vi "AP Main.vi"() -> ()   [LabVIEW 2012]
uses:
  <userlib>/H_Utilities/myDAQ_State.ctl
  Controls/Sheet Colors.ctl
  Controls/Quiz Question.ctl
  Controls/Quiz Solution.ctl
  Spreadsheet/Controls/Spreadsheet Commands.ctl
  Controls/Quiz Mode.ctl
  <vilib>/Utility/sysdir.llb/System Directory Type.ctl
  <vilib>/Platform/browser.llb/Open URL in Default Browser (string).vi
  <userlib>/H_Utilities/myDAQmx/myDAQmx Create Channel/Create myDAQ AI.vi
  <userlib>/H_Utilities/myDAQmx/myDAQmx Create Channel/Create myDAQ DO.vi
  <userlib>/H_Utilities/myDAQmx/myDAQmx Read/myDAQmx Read Analog Value.vi
  <userlib>/H_Utilities/myDAQmx/myDAQmx Read/myDAQmx Read Analog Waveforms.vi
  <userlib>/H_Utilities/myDAQmx/myDAQmxWrite/myDAQmx Write Digital - 1 Chan.vi
panel:
  in  "Quiz Atempts":i32=2
  out "Quiz Questions":i32
  in  "Sheet Colors":T1={"Header Color"=16758784, "Header Font Color"=0, "Font Color"=0, "Clear Color"=16777225, "Alt Clear Color"=15000804}
  in  "AG Page Buttons":enum32{"Page 1", "Page 2", "Page 3", "Page 4"}(radio)
  in  "Exit":bool
  in  "LabVIEW":bool
  in  "Report Issue":bool
  out "Error Out":errorcluster
  out "Event Loop":i32
  out "DAQ Loop":i32
  out "Active State":T2
  in  "AG Pages":enum32{"Page 1", "Page 2", "Page 3", "Page 4"}(tab)
  in  "Explore":bool
  out "Connected":bool
  in  "AG Tab Buttons":enum32{"Tab1", "Tab2", "Tab3"}(radio)
  in  "AG Tabs":enum32{"Tab 1", "Tab 2", "Tab 3"}(tab)
  in  "Configure":bool
  out "Value":dbl(slide) scale=-10.0..10.0
  in  "Measure":bool
  out "Analog Input 0":dbl(knob) scale=-10.0..10.0 scale format="%#.3g"
  in  "DO":bool
  out "Waveform Chart":waveform(dbl)(graph)
  in  "Log to Table":bool
  in  "Event Name":string="Event 1"
  out "Elapsed Time":dbl format="%.2gs"
  in  "Spreadsheet":i32[](listbox)
  in  "Copy":bool
  in  "Clear Sheet":bool
  in  "Save as .csv":bool
  in  "Next Question":bool
  in  "Previous Question":bool
  in  "Grade":bool
  out "Grade String":string
  in  "Problem3":T3={"ProblemNum"=0, "Problem Type"={"Text"="", "Image"=bytes[0], "Text&Image"={"Text (&Image)"="", "Image (&text)"=bytes[0]}}, "Solution Type"={"Numeric"=0.0, "Text"="", "Multi"={"A"=TRUE, "B"=FALSE, "C"=FALSE, "D"=FALSE, "E"=FALSE}, "Radio"=enum."A", "True/False"=enum."True", "Short Answer"=""}, "Answer Color"=0}
  in  "Problem2":T3={"ProblemNum"=0, "Problem Type"={"Text"="", "Image"=bytes[0], "Text&Image"={"Text (&Image)"="", "Image (&text)"=bytes[0]}}, "Solution Type"={"Numeric"=0.0, "Text"="", "Multi"={"A"=TRUE, "B"=FALSE, "C"=FALSE, "D"=FALSE, "E"=FALSE}, "Radio"=enum."A", "True/False"=enum."True", "Short Answer"=""}, "Answer Color"=0}
  in  "Problem1":T3={"ProblemNum"=0, "Problem Type"={"Text"="", "Image"=bytes[0], "Text&Image"={"Text (&Image)"="", "Image (&text)"=bytes[0]}}, "Solution Type"={"Numeric"=0.0, "Text"="", "Multi"={"A"=TRUE, "B"=FALSE, "C"=FALSE, "D"=FALSE, "E"=FALSE}, "Radio"=enum."A", "True/False"=enum."True", "Short Answer"=""}, "Answer Color"=0}
  in  "Problem0":T3={"ProblemNum"=0, "Problem Type"={"Text"="", "Image"=bytes[0], "Text&Image"={"Text (&Image)"="", "Image (&text)"=bytes[0]}}, "Solution Type"={"Numeric"=0.0, "Text"="", "Multi"={"A"=TRUE, "B"=FALSE, "C"=FALSE, "D"=FALSE, "E"=FALSE}, "Radio"=enum."A", "True/False"=enum."True", "Short Answer"=""}, "Answer Color"=0}
  in  "Quiz Scrollbar":i32(c297)
  # "Lab Title"
  # "#update\nIf you change this remeber to set as default"
  # "Getting Started Instructions"
  # "1. Connect myDAQ to this computer.\n\n2. Connect the circuit as shown here."
  # "1. Calibrate your device"
  # "1. Read Signal"
  # "Spreadsheet Title"
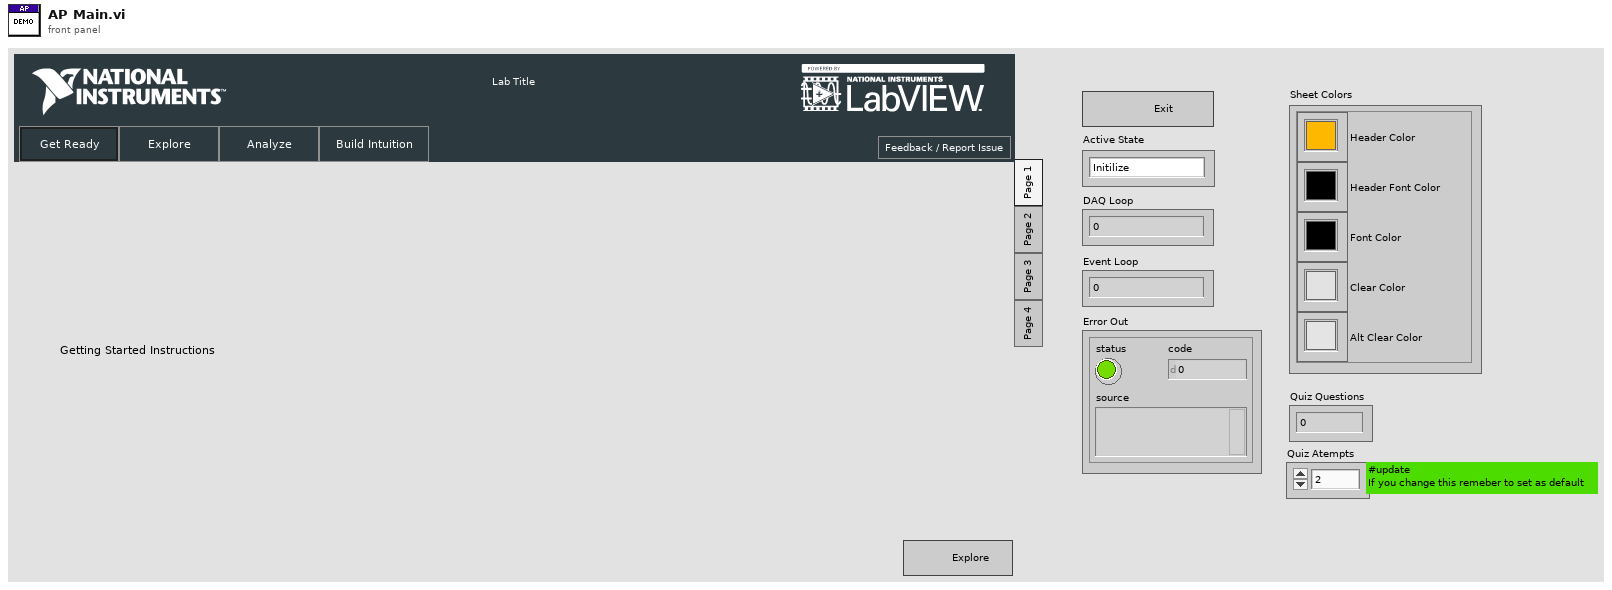
[diagram p1: front panel]
types:
  T1 = typedef "Sheet Colors.ctl" = cluster{"Header Color":u32, "Header Font Color":u32, "Font Color":u32, "Clear Color":u32, "Alt Clear Color":u32}
  T2 = typedef "myDAQ_State.ctl" = enum16{"Initilize", "Connect", "Calibrate", "Communicate", "Wait", "Disconnect", "Error", "Close"}
  T3 = typedef "Quiz Question.ctl" = cluster{"ProblemNum":i32, "Problem Type":cluster{"Text":string, "Image":picture, "Text&Image":cluster{"Text (&Image)":string, "Image (&text)":picture}}, "Solution Type":T4, "Answer Color":u32}
  T4 = typedef "Quiz Solution.ctl" = cluster{"Numeric":dbl, "Text":string, "Multi":cluster{"A":bool, "B":bool, "C":bool, "D":bool, "E":bool}, "Radio":enum32{"No Selection", "A", "B", "C", "D", "E"}, "True/False":enum32{"No Selection", "True", "False"}, "Short Answer":string}
  T5 = enum8{"Enabled", "Disabled", "Disabled and Grayed Out"}
  T6 = typedef "Spreadsheet Commands.ctl" = enum16{"Init", "Clear", "Add", "Mass Add", "Delete Row", "Format Colors"}
  T7 = typedef "Quiz Info.ctl" = cluster{"Question Type":enum16{"Text", "Image", "Text&Image"}, "Solution Type":enum16{"Number", "Text", "MultiChoice", "Radio", "T/F", "Paragraph"}, "Question":cluster{"Text":string, "Image":picture}, "Solution":cluster{"Numeric":cluster{"Min":dbl, "Max":dbl, "Sig Figs":i32, "Sig Figs?":bool}, "Text":string, "True/False":bool, "MultiSelect":cluster{"A":bool, "B":bool, "C":bool, "D":bool, "E":bool}, "MultiText":string[], "Text Case Match":bool}, "Stored Solution":T4, "Button Color":u32}
  T8 = enum32{"invalid app kind", "Development System", "Run Time System", "Student Edition", "Embedded LabVIEW", "Evaluation", "Custom"}
  T9 = typedef "Quiz Mode.ctl" = enum16{"Update", "Store Solution", "Grade"}
  T10 = typedef "System Directory Type.ctl" = i32
  T11 = typedef "LVPoint32TypeDef.ctl" = cluster{"Horizontal":i32, "Vertical":i32}
  T12 = typedef "LVRowAndColumnTypeDef.ctl" = cluster{"Row":i32, "Column":i32}
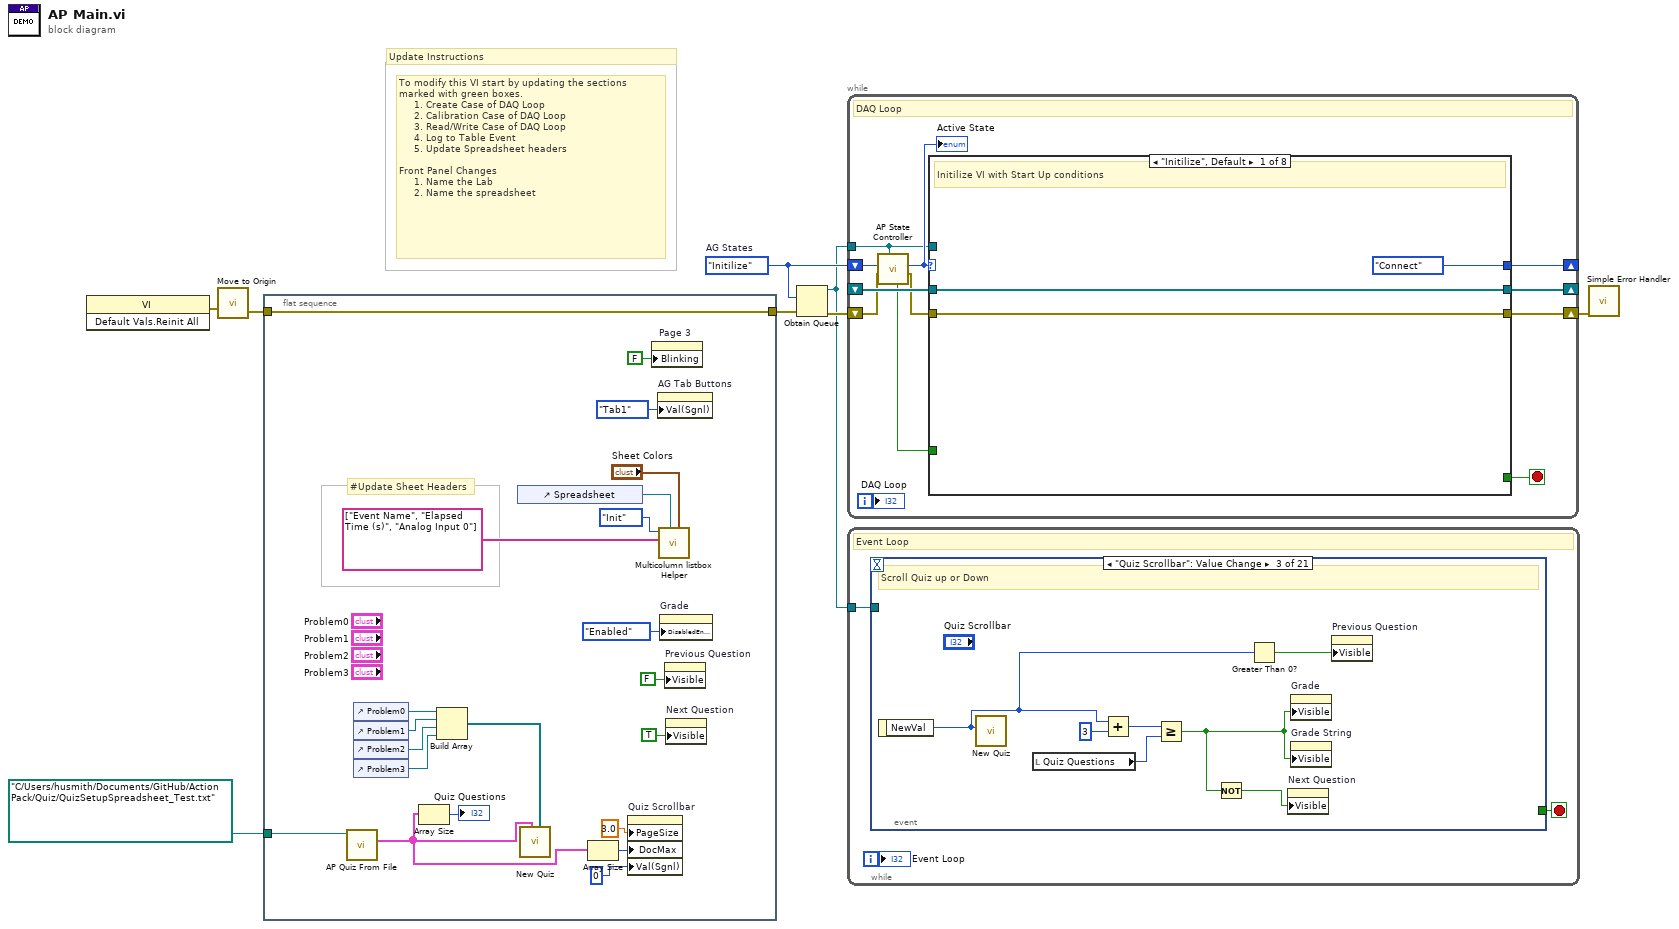
[diagram p0: block diagram]
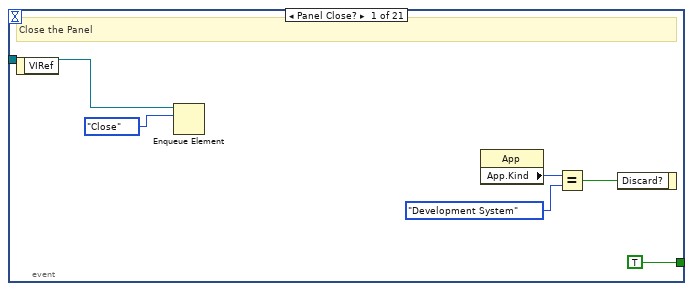
[diagram p2: hidden frame]
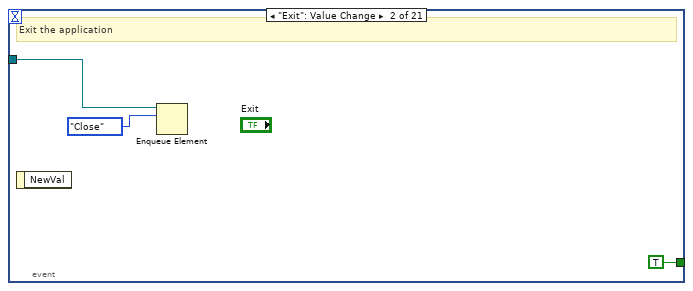
[diagram p3: hidden frame]
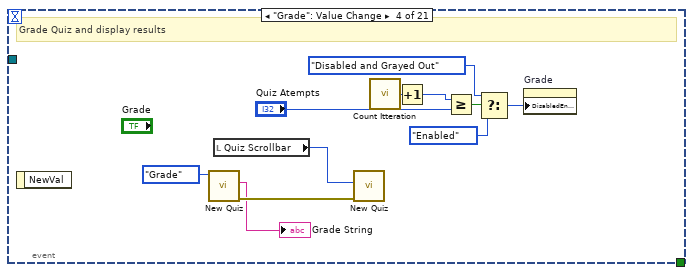
[diagram p4: hidden frame]
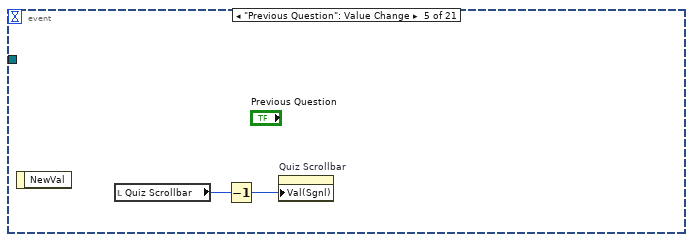
[diagram p5: hidden frame]
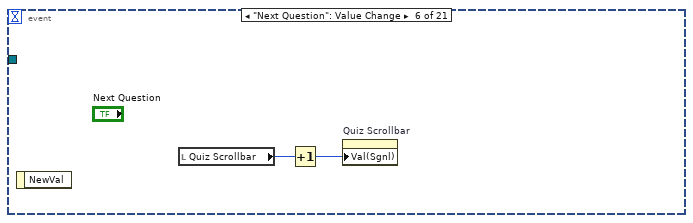
[diagram p6: hidden frame]
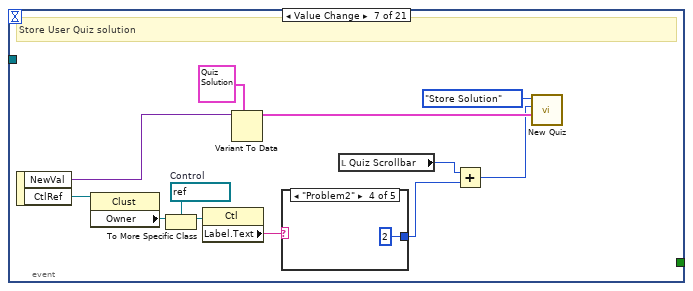
[diagram p7: hidden frame]
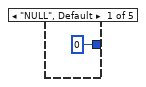
[diagram p8: hidden frame]
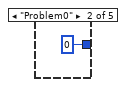
[diagram p9: hidden frame]
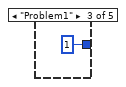
[diagram p10: hidden frame]
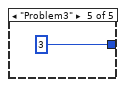
[diagram p11: hidden frame]
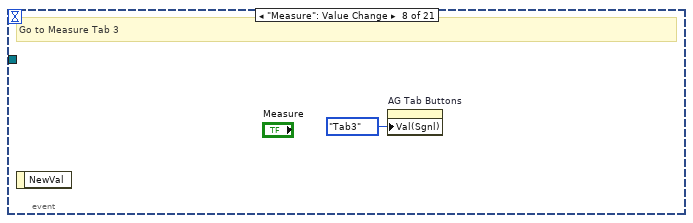
[diagram p12: hidden frame]
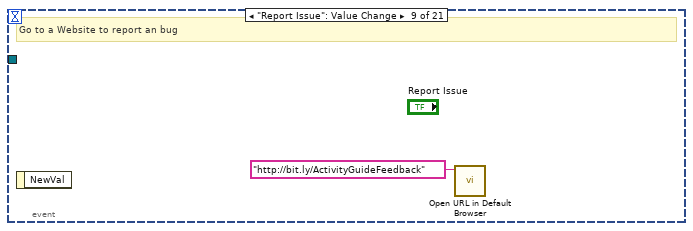
[diagram p13: hidden frame]
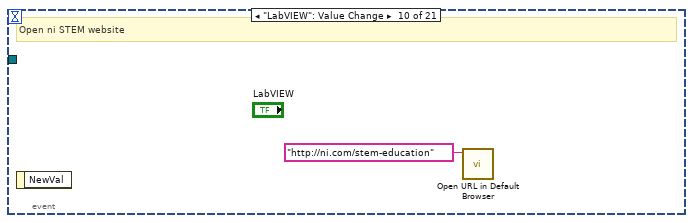
[diagram p14: hidden frame]
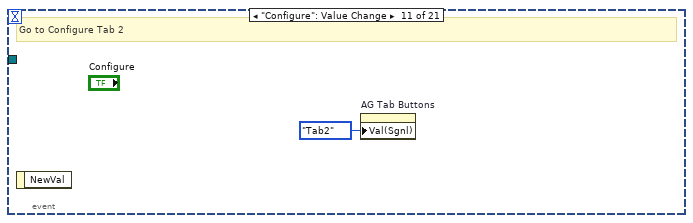
[diagram p15: hidden frame]
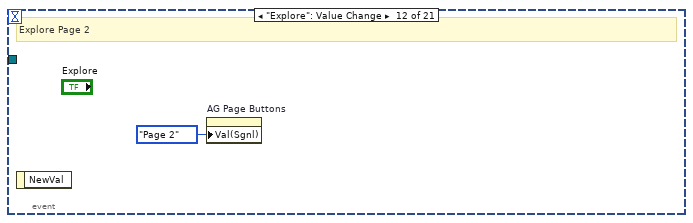
[diagram p16: hidden frame]
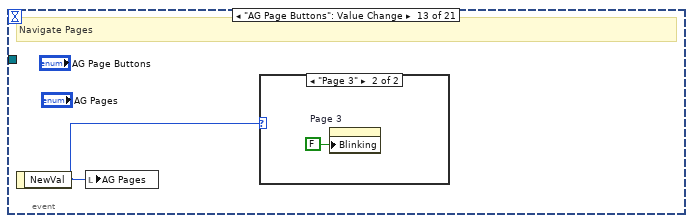
[diagram p17: hidden frame]
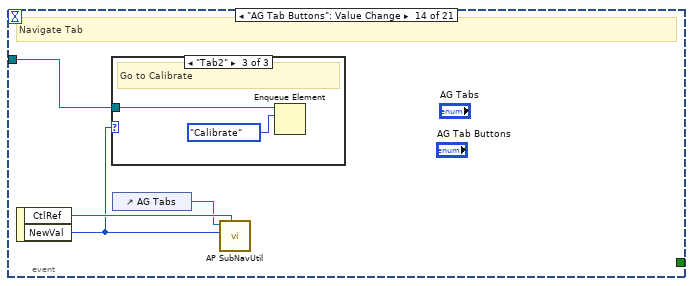
[diagram p19: hidden frame]
diagram:
  w8 = myDAQ_State."Initilize"  # AG States
  # "To modify this VI start by updating the sections marked with green boxes.\n     1. Create Case of DAQ Loop\n     2. Calibration Case of DAQ Loop\n     3. Read/Write Case of DAQ Loop\n     4. Log to Table Event\n     5. Update Spreadsheet headers\n\nFront Panel Changes\n     1. Name the Lab\n     2. Name the spreadsheet"
  # "Update Instructions"
  n1 = invoke class="VI" method="Default Vals.Reinit All"() -> (error out=w2:errorcluster)  [unwired: 3 in, 2 out]
  n2 = call "Move to Origin.vi"("Error In"=w2) -> ("Error Out"=w4:errorcluster)  [unwired: 2 in]
  n3 = flat-sequence {
    tunnel: w4 -> [w29]
    tunnel: [w29] -> w3
    tunnel: path "C:/Users/husmith/Documents/GitHub/Action Pack/Quiz/QuizSetupSpreadsheet_Test.txt" ("file path (dialog if empty)") -> [w14]
    frame #0 {
      # "#Update Sheet Headers"
      n4 = call "AP Quiz From File.vi"("file path (dialog if empty)"=w14) -> ("Question Array Out"=w11:T7[])  [unwired: 8 in, 2 out]
      n5 = control-ref of="Problem0"() -> (w22:refnum<vi>)
      n6 = control-ref of="Problem1"() -> (w21:refnum<vi>)
      n7 = control-ref of="Problem2"() -> (w20:refnum<vi>)
      n8 = control-ref of="Problem3"() -> (w19:refnum<vi>)
      n9 = Array Size(array=w11) -> (size(s)=→"Quiz Questions":i32)
      n10 = Build Array(w22, w21, w20, w19) -> (w18:refnum<vi>[])
      n11 = control-ref of="Spreadsheet"() -> (w24:refnum<vi>)
      n12 = call "New Quiz.vi"("Prob Ref"=w18, "Quiz Data"=w11) -> ()  [unwired: 8 in, 2 out]
      n13 = Array Size(array=w11) -> (size(s)=w17:i32)
      n14 = property on="Quiz Scrollbar" class="Scroll (strict)"("PageSize"=3.0 ("Page Size"), "DocMax"=w17, "Val(Sgnl)"=0 ("Value (Signaling)")) -> ()  [unwired: 2 in, 2 out]
      n15 = property on="Page 3" class="Bool (strict)"("Blinking"=FALSE) -> ()  [unwired: 2 in, 2 out]
      n16 = property on="AG Tab Buttons" class="RadioBtnsControl (strict)"("Val(Sgnl)"=enum32{"Tab1", "Tab2", "Tab3"}."Tab1" ("Value (Signaling)")) -> ()  [unwired: 2 in, 2 out]
      n17 = call "Multicolumn listbox Helper.vi"("Sheet Colors"="Sheet Colors", "Multicolumn Ref"=w24, "Data"=string[] ["Event Name", "Elapsed Time (s)", "Analog Input 0"], "Action (add default)"=Spreadsheet_Commands."Init") -> ()  [unwired: 7 in, 1 out]
      n18 = property on="Grade" class="Bool"("DisabledEnum"=T5."Enabled" ("Disabled")) -> ()  [unwired: 2 in, 2 out]
      n19 = property on="Previous Question" class="Bool"("Visible"=FALSE) -> ()  [unwired: 2 in, 2 out]
      n20 = property on="Next Question" class="Bool"("Visible"=TRUE) -> ()  [unwired: 2 in, 2 out]
    }
  }
  n21 = Obtain Queue(element data type=w8, error in (no error)=w3) -> (queue out=w6:refnum<queue>, error out=w7:errorcluster)  [unwired: 3 in, 1 out]
  n22 = while {
    shift-right: [w41] -> _
    shift-left: _ -> [w39]
    shift-right: [w34] -> _
    shift-left: w8 -> [w38]
    tunnel: w6 -> [w31]
    shift-right: [w40] -> w5
    shift-left: w7 -> [w37]
    i -> [w30]
    stop <- w32 stop-if-true
    # "DAQ Loop"
    n23 = call "AP State Controller.vi"("queue Ref"=w31, "Error In"=w37, "Default State"=w38) -> ("Error Out"=w36:errorcluster, "State Out"=w33:T2, "New State"=w35:bool)  [unwired: 6 in]
    "Active State" <- w33
    n24 = case shown="\"Initilize\", Default" w33 {
      tunnel: [w44 w46 w66 w75 w83 w95 w102 w111] -> w41
      tunnel: [w42 w47 w67 w76 w90 w94 w101 w110] -> w40
      tunnel: w39 -> [w44 w62 w69 w82 w87 w97 w104 w109]
      tunnel: w36 -> [w42 w61 w68 w81 w86 w96 w103 w108]
      tunnel: w35 -> [_ w58 _ _ _ _ _ _]
      tunnel: [myDAQ_State."Connect" ("AG States") w52 myDAQ_State."Calibrate" ("AG States") myDAQ_State."Communicate" ("AG States") w84 myDAQ_State."Wait" ("AG States") w98 myDAQ_State."Close" ("AG States")] -> w34
      tunnel: [_ _ _ _ _ _ _ TRUE] -> w32
      tunnel: w31 -> [_ _ _ _ w91 _ _ _]
      frame "Initilize", Default {
        # "Initilize VI with Start Up conditions"
      }
      frame "Connect" {
        # "#Update Create DAQ Tasks"
        # "Connect to myDAQmx Tasks"
        n25 = call <userlib>:"myDAQmx Safe Clear.vi"("error in (no error)"=w61, "task array in"=w62) -> ("error out"=w60:errorcluster, "task array out"=w63:refnum<k21>[])  [unwired: 8 in]
        n26 = Select(t=u32 0 ("milliseconds to wait"), s=w58, f=u32 250 ("milliseconds to wait")) -> (s? t:f=w55:u32)
        n27 = Wait (ms)(milliseconds to wait=w55) -> ()  [unwired: 1 out]
        n28 = call-poly <userlib>:"myDAQmx Create Channel.vi"("samples per channel(100)"=1, "error in (no error)"=w60, "physical channels (ai0:1)"=tag "myDAQ1/ai0:1", "task array in (none)"=w63) -> ("error out"=w49:errorcluster, "task array out"=w48:refnum<k21>[])  [unwired: 6 in]
        n29 = call-poly <userlib>:"myDAQmx Create Channel.vi"("error in (no error)"=w49, "task array in (none)"=w48) -> ("error out"=w47:errorcluster, "task array out"=w46:refnum<k21>[])  [unwired: 8 in]
        n30 = Unbundle By Name(w47) -> ("status"=w51:bool)
        n31 = Select(t=myDAQ_State."Connect" ("AG States"), s=w47, f=myDAQ_State."Wait" ("AG States")) -> (s? t:f=w52:T2)
        n32 = Not(x=w51) -> (.not. x?=→"Connected":bool)
      }
      frame "Calibrate" {
        # "#Update Calibrate"
        # "Calibrate DAQ Tasks"
        n33 = call-poly <userlib>:"myDAQmx Read.vi"("error in (no error)"=w68, "task array in"=w69) -> ("error out"=w67:errorcluster, "value 0"=→"Value":dbl, "task array out"=w66:refnum<k21>[])  [unwired: 6 in, 1 out]
        n34 = Wait Until Next ms Multiple(millisecond multiple=u32 20) -> ()  [unwired: 1 out]
      }
      frame "Communicate" {
        # "#Update Read /Write DAQ & Analyze"
        # "Read / Write myDAQmx Tasks Here & perform analysis"
        n35 = call-poly <userlib>:"myDAQmx Read.vi"("error in (no error)"=w81, "# of samples per channel (-1)"=1, "task array in"=w82) -> ("error out"=w77:errorcluster, "waveform 1"=w72:waveform(dbl), "task array out"=w78:refnum<k21>[])  [unwired: 2 in, 4 out]
        "Waveform Chart" <- w72
        "Analog Input 0" <- w72
        n36 = call "Extract M-S from Timestamp.vi"("Waveform"=w72) -> ("Elapsed Time (s)"=→"Elapsed Time":dbl)  [unwired: 9 in, 1 out]
        n37 = call-poly <userlib>:"myDAQmx Write.vi"("error in (no error)"=w77, "value (F)"="DO", "task array in"=w78) -> ("error out"=w76:errorcluster, "task array out"=w75:refnum<k21>[])  [unwired: 7 in]
        n38 = Wait Until Next ms Multiple(millisecond multiple=u32 20) -> ()  [unwired: 1 out]
      }
      frame "Wait" {
        # "Wait for New Command in State Queue"
        n39 = call <userlib>:"myDAQmx Stop Task.vi"("error In"=w86, "task array in"=w87) -> ("Error Out"=w88:errorcluster, "task array out"=w89:refnum<k21>[])  [unwired: 8 in]
        n40 = call <userlib>:"myDAQmx Handle Errors.vi"("Error In"=w88, "Task Array In"=w89) -> ("Error Out"=w85:errorcluster, "Task Array Out"=w83:refnum<k21>[])  [unwired: 6 in, 2 out]
        n41 = Preview Queue Element(queue=w91, error in (no error)=w85) -> (element=w84:T2, error out=w90:errorcluster)  [unwired: 1 in, 2 out]
      }
      frame "Disconnect" {
        # "Disconnect from DAQ device"
        n42 = call <userlib>:"myDAQmx Safe Clear.vi"("error in (no error)"=w96, "task array in"=w97) -> ("error out"=w94:errorcluster, "task array out"=w95:refnum<k21>[])  [unwired: 8 in]
        n43 = local write "Connected"(FALSE ("Connected")) -> ()
      }
      frame "Error" {
        # "Error Found, Handle and Continue"
        n44 = call <userlib>:"myDAQmx Handle Errors.vi"("Error In"=w103, "Task Array In"=w104) -> ("Error Out"=w101:errorcluster, "Task Array Out"=w102:refnum<k21>[])  [unwired: 6 in, 2 out]
        n45 = Select(t=myDAQ_State."Close" ("AG States"), s=w101, f=myDAQ_State."Connect" ("AG States")) -> (s? t:f=w98:T2)
        "Error Out" <- w103
      }
      frame "Close" {
        n46 = local write "Connected"(FALSE ("Connected")) -> ()
        n47 = property on="Exit" class="Bool (strict)"("Val(Sgnl)"=TRUE ("Connected")) -> ()  [unwired: 2 in, 2 out]
        n48 = call <userlib>:"myDAQmx Safe Clear.vi"("error in (no error)"=w108, "task array in"=w109) -> ("error out"=w110:errorcluster, "task array out"=w111:refnum<k21>[])  [unwired: 8 in]
      }
    }
    "DAQ Loop" <- w30
  }
  n49 = while {
    tunnel: w6 -> [w115]
    i -> [w113]
    stop <- w114 stop-if-true
    # "Event Loop"
    n50 = event shown="[2] \"Quiz Scrollbar\": Value Change" {
      selector: _ -> [_ _ _ _ _ _ _ _ _ _ _ _ _ _ _ _ _ _ _ _ _]
      dyn-events: _ -> [_ _ _ _ _ _ _ _ _ _ _ _ _ _ _ _ _ _ _ _ _]
      timeout: _ -> [_ _ _ _ _ _ _ _ _ _ _ _ _ _ _ _ _ _ _ _ _]
      tunnel: w115 -> [w121 w124 _ _ _ _ _ _ _ _ _ _ _ w171 _ _ _ _ _ _ _]
      tunnel: [TRUE TRUE _ _ _ _ _ _ _ _ _ _ _ _ _ _ _ _ _ _ _] -> w114
      event Panel Close? {
        # "Close the Panel"
        n51 = event-data() -> ()  [unwired: 1 in, 1 out]
        n52 = Enqueue Element(queue=w121, element=myDAQ_State."Close") -> ()  [unwired: 2 in, 3 out]
        n53 = property class="App"() -> ("App.Kind"=w118:T8)  [unwired: 2 in, 2 out]
        n54 = Equal?(x=w118, y=T8."Development System" ("Application:Kind")) -> (x = y?=w116:bool)
        n55 = event-data("Discard?"=w116) -> ()  [unwired: 1 in, 1 out]
      }
      event "Exit": Value Change {
        # "Exit the application"
        n56 = event-data() -> ()  [unwired: 1 in, 1 out]
        n57 = Enqueue Element(queue=w124, element=myDAQ_State."Close") -> ()  [unwired: 2 in, 3 out]
      }
      event "Quiz Scrollbar": Value Change {
        # "Scroll Quiz up or Down"
        n58 = event-data() -> ("NewVal"=w128:i32)  [unwired: 1 in]
        n59 = call "New Quiz.vi"("Index"=w128) -> ()  [unwired: 9 in, 2 out]
        n60 = local read "Quiz Questions"() -> (w129:i32)
        n61 = Add(x=w128, y=3) -> (x+y=w130:i32)
        n62 = Greater Or Equal?(x=w130, y=w129) -> (x >= y?=w126:bool)
        n63 = Not(x=w126) -> (.not. x?=w125:bool)
        n64 = Greater Than 0?(x=w128) -> (x > 0?=w127:bool)
        n65 = property on="Next Question" class="Bool"("Visible"=w125) -> ()  [unwired: 2 in, 2 out]
        n66 = property on="Grade" class="Bool"("Visible"=w126) -> ()  [unwired: 2 in, 2 out]
        n67 = property on="Grade String" class="Str"("Visible"=w126) -> ()  [unwired: 2 in, 2 out]
        n68 = property on="Previous Question" class="Bool"("Visible"=w127) -> ()  [unwired: 2 in, 2 out]
      }
      event "Grade": Value Change {
        # "Grade Quiz and display results"
        n69 = event-data() -> ()  [unwired: 1 in, 1 out]
        n70 = call "New Quiz.vi"("Mode"=Quiz_Mode."Grade") -> ("Error Out"=w141:errorcluster, "Grade String"=→"Grade String":string)  [unwired: 9 in]
        n71 = local read "Quiz Scrollbar"() -> (w140:i32)
        n72 = call "New Quiz.vi"("Error In"=w141, "Index"=w140) -> ()  [unwired: 8 in, 2 out]
        n73 = call "Count Itteration.vi"() -> ("Itteration"=w138:i32)  [unwired: 7 in, 1 out]
        n74 = Increment(x=w138) -> (x+1=w132:i32)
        n75 = Greater Or Equal?(x=w132, y="Quiz Atempts") -> (x >= y?=w136:bool)
        n76 = Select(t=T5."Disabled and Grayed Out" ("Disabled"), s=w136, f=T5."Enabled" ("Disabled")) -> (s? t:f=w133:T5)
        n77 = property on="Grade" class="Bool"("DisabledEnum"=w133) -> ()  [unwired: 2 in, 2 out]
      }
      event "Previous Question": Value Change {
        n78 = event-data() -> ()  [unwired: 1 in, 1 out]
        n79 = local read "Quiz Scrollbar"() -> (w144:i32)
        n80 = Decrement(x=w144) -> (x-1=w143:i32)
        n81 = property on="Quiz Scrollbar" class="Scroll (strict)"("Val(Sgnl)"=w143) -> ()  [unwired: 2 in, 2 out]
      }
      event "Next Question": Value Change {
        n82 = event-data() -> ()  [unwired: 1 in, 1 out]
        n83 = local read "Quiz Scrollbar"() -> (w146:i32)
        n84 = Increment(x=w146) -> (x+1=w145:i32)
        n85 = property on="Quiz Scrollbar" class="Scroll (strict)"("Val(Sgnl)"=w145) -> ()  [unwired: 2 in, 2 out]
      }
      event Value Change {
        w152 = refnum<vi> refnum  # Control
        # "Store User Quiz solution"
        n86 = event-data() -> ("NewVal"=w158:variant, "CtlRef"=w155:refnum<vi>)  [unwired: 1 in]
        n87 = property class="Clust"(reference=w155) -> ("Owner"=w154:refnum<vi>)  [unwired: 1 in, 2 out]
        n88 = To More Specific Class(target class=w152, reference=w154) -> (specific class reference=w153:refnum<vi>)  [unwired: 1 in, 1 out]
        n89 = property class="Ctl"(reference=w153) -> ("Label.Text"=w151:string)  [unwired: 1 in, 2 out]
        n90 = Variant To Data(type=T4 {"Numeric"=0.0, "Text"="", "Multi"={"A"=FALSE, "B"=FALSE, "C"=FALSE, "D"=FALSE, "E"=FALSE}, "Radio"=enum."No Selection", "True/False"=enum."No Selection", "Short Answer"=""} ("Quiz Solution"), Variant=w158) -> (data=w156:T4)  [unwired: 1 in, 1 out]
        n91 = case shown="\"Problem2\"" w151 {
          tunnel: [0 0 1 2 3] -> w149
          frame "NULL", Default {
          }
          frame "Problem0" {
          }
          frame "Problem1" {
          }
          frame "Problem2" {
          }
          frame "Problem3" {
          }
        }
        n92 = local read "Quiz Scrollbar"() -> (w150:i32)
        n93 = Add(x=w150, y=w149) -> (x+y=w148:i32)
        n94 = call "New Quiz.vi"("Quiz Solution"=w156, "Index"=w148, "Mode"=Quiz_Mode."Store Solution") -> ()  [unwired: 7 in, 2 out]
      }
      event "Measure": Value Change {
        # "Go to Measure Tab 3"
        n95 = event-data() -> ()  [unwired: 1 in, 1 out]
        n96 = property on="AG Tab Buttons" class="RadioBtnsControl (strict)"("Val(Sgnl)"=enum32{"Tab1", "Tab2", "Tab3"}."Tab3" ("Value (Signaling)")) -> ()  [unwired: 2 in, 2 out]
      }
      event "Report Issue": Value Change {
        # "Go to a Website to report an bug"
        n97 = event-data() -> ()  [unwired: 1 in, 1 out]
        n98 = call-poly <vilib>:"Open URL in Default Browser.vi"("URL"="http://bit.ly/ActivityGuideFeedback") -> ()  [unwired: 5 in, 2 out]
      }
      event "LabVIEW": Value Change {
        # "Open ni STEM website"
        n99 = event-data() -> ()  [unwired: 1 in, 1 out]
        n100 = call-poly <vilib>:"Open URL in Default Browser.vi"("URL"="http://ni.com/stem-education") -> ()  [unwired: 5 in, 2 out]
      }
      event "Configure": Value Change {
        # "Go to Configure Tab 2"
        n101 = event-data() -> ()  [unwired: 1 in, 1 out]
        n102 = property on="AG Tab Buttons" class="RadioBtnsControl (strict)"("Val(Sgnl)"=enum32{"Tab1", "Tab2", "Tab3"}."Tab2" ("Value (Signaling)")) -> ()  [unwired: 2 in, 2 out]
      }
      event "Explore": Value Change {
        # "Explore Page 2"
        n103 = event-data() -> ()  [unwired: 1 in, 1 out]
        n104 = property on="AG Page Buttons" class="RadioBtnsControl (strict)"("Val(Sgnl)"=enum32{"Page 1", "Page 2", "Page 3", "Page 4"}."Page 2" ("Value (Signaling)")) -> ()  [unwired: 2 in, 2 out]
      }
      event "AG Page Buttons": Value Change {
        # "Navigate Pages"
        n105 = event-data() -> ("NewVal"=w169:enum32{"Page 1", "Page 2", "Page 3", "Page 4"})  [unwired: 1 in]
        n106 = local write "AG Pages"(w169) -> ()
        n107 = case shown="\"Page 3\"" w169 {
          frame "Page 1", Default {
          }
          frame "Page 3" {
            n108 = property on="Page 3" class="Bool (strict)"("Blinking"=FALSE) -> ()  [unwired: 2 in, 2 out]
          }
        }
      }
      event "AG Tab Buttons": Value Change {
        # "Navigate Tab"
        n109 = event-data() -> ("CtlRef"=w174:refnum<vi>, "NewVal"=w172:enum32{"Tab1", "Tab2", "Tab3"})  [unwired: 1 in]
        n110 = case shown="\"Tab2\"" w172 {
          tunnel: w171 -> [_ w175 w177]
          frame "Tab1", Default {
          }
          frame "Tab3" {
            # "Run DAQ Device"
            n111 = Enqueue Element(queue=w175, element=myDAQ_State."Communicate") -> ()  [unwired: 2 in, 3 out]
          }
          frame "Tab2" {
            # "Go to Calibrate"
            n112 = Enqueue Element(queue=w177, element=myDAQ_State."Calibrate") -> ()  [unwired: 2 in, 3 out]
          }
        }
        n113 = control-ref of="AG Tabs"() -> (w173:refnum<vi>)
        n114 = call "AP SubNavUtil.vi"("Progress Ref"=w174, "NewVal"=w172, "Tab Ref"=w173) -> ()  [unwired: 8 in, 1 out]
      }
      event "Spreadsheet": Double Click {
        # "#TODO fix number based Alphabetizing"
        # "Sort by Column"
        n115 = event-data() -> ("CtlRef"=w180:refnum<vi>)  [unwired: 1 in]
        n116 = invoke class="MCListbox (strict)" method="Get Clicked Col Hdr"(reference=w180) -> (reference out=w182:refnum<vi>, error out=w181:errorcluster, "Get Clicked Column Header"=w179:i32)  [unwired: 2 in]
        n117 = call "Sort Spreadsheet by Column.vi"("Error In"=w181, "Column Number"=w179, "Ref In"=w182) -> ()  [unwired: 8 in, 1 out]
      }
      event "Copy": Value Change {
        # "Copy Spreadhseet Data to the clipboard"
        n118 = event-data() -> ()  [unwired: 1 in, 1 out]
        n119 = property on="Spreadsheet" class="MCListbox (strict)"() -> (error out=w183:errorcluster, "ColHdrString"=w186:string[], "ItemNames"=w187:string[][])  [unwired: 2 in, 1 out]
        n120 = Build Array (concatenate)(w186, w187) -> (w188:string[][])
        n121 = Array To Spreadsheet String(array=w188, 3:"" ("format string")) -> (spreadsheet string=w185:string)  [unwired: 1 in]
        n122 = invoke class="App" method="Clipboard.Write"(error in=w183, "Param 0"=w185) -> ()  [unwired: 2 in, 4 out]
      }
      event "Log to Table": Value Change {
        # "#Update Sheet Data"
        # "Log DAQ data to Spreadsheet"
        n123 = event-data() -> ()  [unwired: 1 in, 1 out]
        n124 = local read "Analog Input 0"() -> (w191:dbl)
        n125 = local read "Elapsed Time"() -> (w194:dbl)
        n126 = Number To Fractional String(number=w194, precision (6)=i16 3) -> (F-format string=w195:string)  [unwired: 2 in]
        n127 = Number To Fractional String(number=w191, precision (6)=i16 2) -> (F-format string=w198:string)  [unwired: 2 in]
        n128 = call "Increment Name.vi"("Sample Name"="Event Name") -> ("Sample Name 2"=w193:string)
        n129 = local write "Event Name"(w193) -> ()
        n130 = Build Array("Event Name", w195, w198) -> (w192:string[])
        n131 = call "Multicolumn listbox Helper.vi"("Data"=w192, "Action (add default)"=Spreadsheet_Commands."Add") -> ()  [unwired: 9 in, 1 out]
        n132 = property on="Page 3" class="Bool (strict)"("Blinking"=TRUE) -> ()  [unwired: 2 in, 2 out]
      }
      event "Save as .csv": Value Change {
        w201 = T10 1 items=["User Home"=0, "User Desktop"=1, "User Documents"=2, "User Application Data"=3, "User Preferences"=4, "User Temporary"=5, "Public Documents"=6, "Public Application Data"=7, "Public Preferences"=8, "Public Cache"=13, "System Core Libraries"=9, "System Installed Libraries"=10, "Application Files"=11, "Boot Volume Root"=12] ("system directory type")
        # "Save Spreadsheet at .csv file"
        n133 = event-data() -> ()  [unwired: 1 in, 1 out]
        n134 = call <vilib>:"Get System Directory.vi"("system directory type"=w201) -> ("system directory"=w213:path)  [unwired: 10 in]
        n135 = call "File Dialog"("start path"=w213, "prompt"="Please select a file to save your data.", "default name"="MySpreadsheet", "pattern (all files)"="*.csv", "pattern label"="Comma Seperated Value Files") -> ("selected path"=w203:path, "error out"=w206:errorcluster)  [unwired: 7 in, 2 out]
        n136 = Strip Path(path=w203) -> (name=w210:string)  [unwired: 1 out]
        n137 = Match Pattern(string=w210, regular expression="[.]") -> (after substring=w209:string)  [unwired: 1 in, 3 out]
        n138 = Equal?(x=w209, y="csv") -> (x = y?=w204:bool)
        n139 = Select(t=w206, s=w204, f=errorcluster {"status"=TRUE, "code"=25, "source"=""}) -> (s? t:f=w202:errorcluster)
        n140 = Unbundle By Name(w202) -> ("code"=w207:i32)
        n141 = case shown="0" w207 {
          tunnel: w203 -> [w224 _ _]
          tunnel: w202 -> [w217 _ _]
          frame 0 {
            # "Only Write File If No Error"
            n142 = property on="Spreadsheet" class="MCListbox (strict)"(error in=w217) -> (error out=w218:errorcluster, "ColHdrString"=w219:string[], "ItemNames"=w220:string[][])  [unwired: 1 in, 1 out]
            n143 = Build Array (concatenate)(w219, w220) -> (w221:string[][])
            n144 = Array To Spreadsheet String(delimiter (Tab)=",", array=w221, 3:"" ("format string")) -> (spreadsheet string=w216:string)
            n145 = Write to Text File(file (use dialog)=w224, text=w216, error in=w218) -> ()  [unwired: 1 in, 3 out]
          }
          frame 25 {
            # "Selected non CSV File"
            n146 = One Button Dialog(message="Please select a .csv file. Once you save the file you can open it up in Microsoft Excel or other spreadsheet applications. ", button name ("OK")="OK" ("format string")) -> ()  [unwired: 1 out]
          }
          frame 43, Default {
            # "Cancel File Dialog"
            n147 = One Button Dialog(message="File Not Saved") -> ()  [unwired: 1 in, 1 out]
          }
        }
      }
      event "Spreadsheet": Shortcut Menu Selection (User) {
        # "Delete a Row using the right-click options"
        n148 = event-data() -> ("CtlRef"=w228:refnum<vi>, "ItemPath"=w230:string, "Coords"=w229:T11)  [unwired: 1 in]
        n149 = case shown="\"Delete_this_Row\"" w230 {
          tunnel: w229 -> [_ w237]
          tunnel: w228 -> [_ w233]
          frame "NULL", Default {
          }
          frame "Delete_this_Row" {
            n150 = invoke on="Invoke Node" class="MCListbox (strict)" method="Point To Row Column"(reference=w233, "Point"=w237) -> (reference out=w232:refnum<vi>, error out=w235:errorcluster, "CellPosition"=w236:T12)  [unwired: 5 in, 4 out]
            n151 = Unbundle By Name(w236) -> ("Row"=w231:i32)
            n152 = call "Multicolumn listbox Helper.vi"("Row to Delete"=w231, "Multicolumn Ref"=w232, "Error In"=w235, "Action (add default)"=Spreadsheet_Commands."Delete Row") -> ()  [unwired: 7 in, 1 out]
          }
        }
      }
      event Value Change {
        n153 = event-data() -> ()  [unwired: 1 in, 1 out]
      }
      event "Clear Sheet": Value Change {
        # "Clear the Spreadsheet"
        n154 = event-data() -> ()  [unwired: 1 in, 1 out]
        n155 = Two Button Dialog(message="Are you sure you want to clear the Log, all data on this spreadsheet will be lost.", 2:"Yes" ("T button name (\"OK\")")) -> (T button?=w240:bool)  [unwired: 1 in]
        n156 = case shown="True" w240 {
          frame False {
          }
          frame True {
            n157 = call "Multicolumn listbox Helper.vi"("Action (add default)"=Spreadsheet_Commands."Clear") -> ()  [unwired: 10 in, 1 out]
          }
        }
      }
    }
    "Event Loop" <- w113
  }
  n158 = call <vilib>:"Simple Error Handler.vi"("error in (no error)"=w5) -> ()  [unwired: 4 in, 5 out]
